vi "niRFSTS Digitizer Close.vi"(10 "Instrument Type Id":string, 11 "TSM Context":T1) -> (0 "error out":errorcluster)   [LabVIEW 2014]
uses:
  <vilib>/NI_TestStand_SemiconductorModule/NI_TestStand_Semiconductor_Module.lvlibp/PinMap/General/SemiconductorModuleContext.ctl
  <vilib>/NI_TestStand_SemiconductorModule/NI_TestStand_Semiconductor_Module.lvlibp
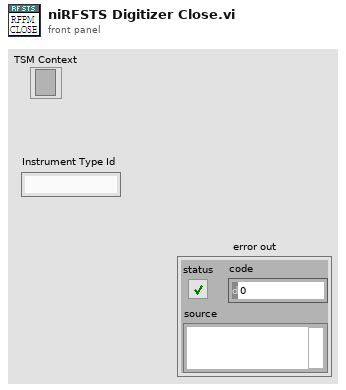
[diagram p1: front panel]
types:
  T1 = typedef "NI_TestStand_Semiconductor_Module.lvlibp/SemiconductorModuleContext.ctl" = refnum<k7>
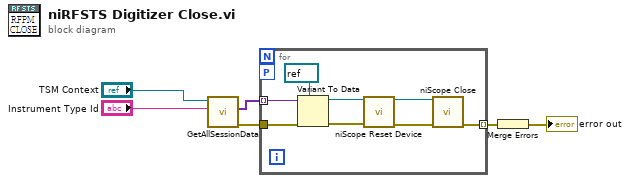
[diagram p0: block diagram]
diagram:
  n1 = call <vilib>:"GetAllSessionData.vi"("Instrument Type Id"="Instrument Type Id", "Semiconductor Module Context"="TSM Context") -> ("error out"=w4:errorcluster, "Session Data"=w3:variant[])  [unwired: 5 in, 3 out]
  n2 = for {
    workers-P: _ -> [_]
    tunnel: [w14] -> w6 mode=indexing
    tunnel: w4 -> [w13]
    tunnel: w3 -> [w12] mode=indexing
    n3 = Variant To Data(error in=w13, type=refnum<k15> refnum ("instrument handle"), Variant=w12) -> (data=w10:refnum<k15>, error out=w8:errorcluster)
    n4 = call <instrlib>:"niScope Reset Device.vi"("instrument handle"=w10, "error in"=w8) -> ("instrument handle out"=w9:refnum<k15>, "error out"=w7:errorcluster)  [unwired: 12 in]
    n5 = call <instrlib>:"niScope Close.vi"("instrument handle"=w9, "error in"=w7) -> ("error out"=w14:errorcluster)  [unwired: 13 in]
  }
  n6 = Merge Errors(w6) -> (→"error out":errorcluster)
